vi "hardware_initialize_hardware.vi"(8 "error in (no error)":errorcluster, 11 "thorlabs_FW102C in":refnum<class "thorlabs_FW102C.lvclass">) -> (0 "error out":errorcluster, 3 "thorlabs_FW102C out":refnum<class "thorlabs_FW102C.lvclass">)   [LabVIEW 2015, in "thorlabs_FW102C.lvclass"]
uses:
  thorlabs_FW102C.lvclass
  thorlabs_FW102C.lvclass/thorlabs_FW102C.ctl
  Thorlabs_FW102C.lvlib
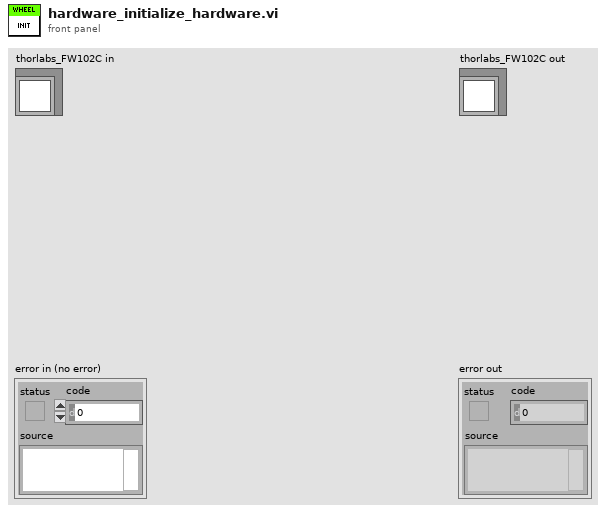
[diagram p1: front panel]
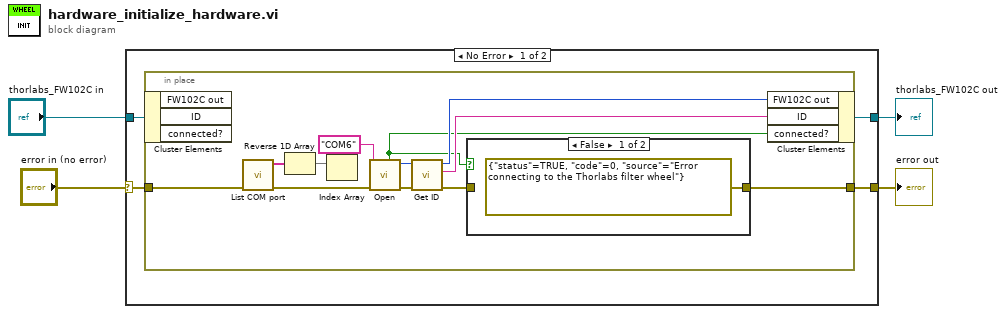
[diagram p0: block diagram]
diagram:
  n1 = case shown="No Error" "error in (no error)" {
    selector: "error in (no error)" -> [w7 w23]
    tunnel: "thorlabs_FW102C in" -> [w8 w24]
    tunnel: [w6 w23] -> w2
    tunnel: [w5 w24] -> w1
    frame No Error {
      n2 = in-place {
        in-place-border: w7 -> [w15]
        in-place-border: [w10] -> w6
        n3 = in-place-cluster #1(w8) -> ()  [unwired: 3 out]
        n4 = call "List COM port.vi"("error in (no error)"=w15) -> ("error out"=w16:errorcluster, "COM Ports"=w18:string[])  [unwired: 9 in]
        n5 = Reverse 1D Array(array=w18) -> (reversed array=w17:string[])
        n6 = Index Array(array=w17) -> ()  [unwired: 1 in, 1 out]
        n7 = call "Open.vi"("error in (no error)"=w16, "Serial Port"="COM6") -> ("error out"=w19:errorcluster, "FW102C out"=w20:i32, "Connected?"=w12:bool)  [unwired: 7 in]
        n8 = call "Get ID.vi"("error in (no error)"=w19, "FW102C in"=w20) -> ("error out"=w11:errorcluster, "ID"=w13:string, "FW102C out"=w14:i32)  [unwired: 7 in]
        n9 = case shown="False" w12 {
          tunnel: w11 -> [_ w22]
          tunnel: [errorcluster {"status"=TRUE, "code"=0, "source"="Error connecting to the Thorlabs filter wheel"} ("error out") w22] -> w10
          frame False {
          }
          frame True {
          }
        }
        n10 = in-place-cluster #1("FW102C out"=w14, "ID"=w13, "connected?"=w12) -> (w5:refnum<class "thorlabs_FW102C.lvclass">)
      }
    }
    frame Error {
    }
  }
  "error out" <- w2
  "thorlabs_FW102C out" <- w1
